vi "test_Set and Get 9228.vi"(8 "error in (no error)":errorcluster, 11 "TestCase in":refnum<class "Scan Engine Scripting API Custom Device Unit Tests.lvclass">) -> (0 "error out":errorcluster, 3 "TestCase out":refnum<class "Scan Engine Scripting API Custom Device Unit Tests.lvclass">)   [LabVIEW 2017, in "Scan Engine Scripting API Custom Device Unit Tests.lvclass"]
uses:
  Scan Engine Scripting API Custom Device Unit Tests.lvclass
  Scan Engine Scripting API Custom Device Unit Tests.lvclass/Scan Engine Scripting API Custom Device Unit Tests.ctl
  8367f121-9304-47f9-89de-0b88beeae42b.vi
  Utility/Set Error.vi
  <vilib>/Utility/error.llb/Clear Errors.vi
  Scripting/Modules/NI 9228/NI 9228.lvclass
  C:/Users/nitest/Documents/niveristand-scan-engine-ethercat-custom-device/Custom Device Source/Scripting/Modules/Module/Module.lvclass
  Modules.lvlibp/SD Module/SD Module.lvclass
  C:/Users/nitest/Documents/niveristand-scan-engine-ethercat-custom-device/Custom Device Source/Modules.lvlibp/RSI Module/RSI Module.lvclass
  Scripting/Modules/NI 9224/NI 9224.lvclass
  Modules.lvlibp/RSI Module/Read Module Page Property.vi
  Modules.lvlibp/RSI Module/Read Model.vi
  Scripting/Utility/Convert Module Model to Module Class.vi
  Modules.lvlibp/SD Module/Read DIO mode.vi
  Modules.lvlibp/RSI Module/Read Channels.vi
  Scripting/Utility/Convert to DI Module.vi
  Scripting/Utility/Convert to DO Module.vi
  Scripting/Utility/Convert to CI PWM Module.vi
  Scripting/Utility/Convert to CDO Module.vi
  Scripting/Utility/Convert to PWM Module.vi
  Globals/Error Strings.vi
  Scripting/Utility/Convert to AI Vrms Module.vi
  Scripting/Utility/Convert to AI Module.vi
  Scripting/Modules/Module/Module.lvclass
  Modules.lvlibp/9224/9224.lvclass
  <vilib>/addons/_JKI Toolkits/VI Tester/TestCase.llb/TestCase.lvclass
  Scripting/Scan Engine Scripting.lvlib
  C:/Program Files (x86)/National Instruments/LabVIEW 2017/vi.lib/addons/_JKI Toolkits/VI Tester/TestCase.llb/TestCase.lvclass
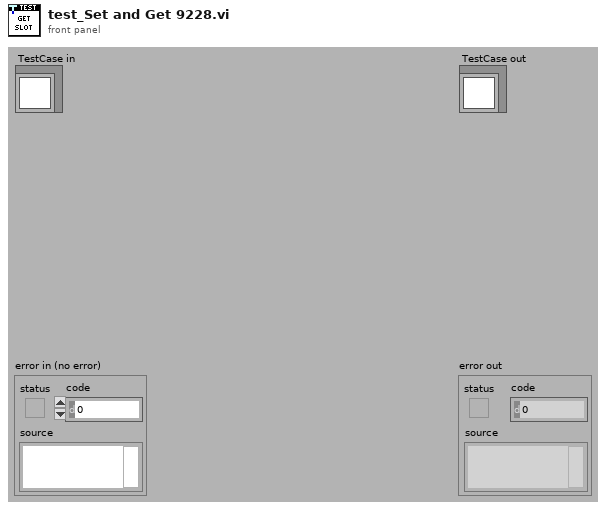
[diagram p1: front panel]
types:
  T1 = typedef "Custom Device API.lvlib/Custom Device Item Ref.ctl" = u64
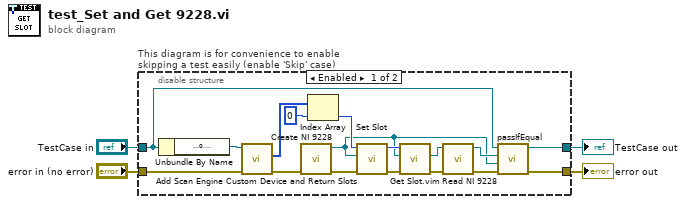
[diagram p0: block diagram]
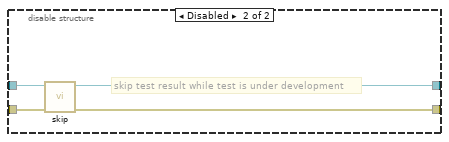
[diagram p2: hidden frame]
diagram:
  n1 = disable-structure "This diagram is for convenience to enable skipping a test easily (enable 'Skip' case)" shown="Enabled" {
    disable-tunnel: "TestCase in" -> [w18 w25]
    disable-tunnel: [w12 w23] -> w1
    disable-tunnel: [w16 w24] -> w3
    disable-tunnel: "error in (no error)" -> [w5 w22]
    frame Enabled {
      n2 = Unbundle By Name(w18) -> ("target ref"=w8:refnum<k24>)
      n3 = call "Add Scan Engine Custom Device and Return Slots.vi"("error in"=w5, "target ref in"=w8) -> ("error out"=w6:errorcluster, "slot refs"=w7:T1[])  [unwired: 7 in, 1 out]
      n4 = call "Create NI 9228.vi"("error in"=w6) -> ("error out"=w17:errorcluster, "NI 9228 out"=w11:refnum<class "NI 9228.lvclass">)  [unwired: 9 in]
      n5 = Index Array(array=w7, index=0) -> (element=w21:T1)
      n6 = call "Set Slot.vi"("error in"=w17, "module"=w11, "slot ref in"=w21) -> ("error out"=w19:errorcluster, "slot ref out"=w13:T1)  [unwired: 7 in]
      n7 = call "Get Slot.vim"("error in"=w19, "module in"=w11, "slot ref in"=w13) -> ("error out"=w9:errorcluster, "module"=w10:refnum<class "NI 9228.lvclass">)  [unwired: 5 in, 2 out]
      n8 = call "Read NI 9228.vi"("error in"=w9, "NI 9228 in"=w10) -> ("error out"=w14:errorcluster, "NI 9228 out"=w15:refnum<class "NI 9228.lvclass">)  [unwired: 6 in, 2 out]
      n9 = call-dynamic "passIfEqual.vi"("error in (no error)"=w14, "y"=w11, "x"=w15, "TestCase in"=w18) -> ("error out"=w16:errorcluster, "TestCase out"=w12:refnum<class "Scan Engine Scripting API Custom Device Unit Tests.lvclass">)  [unwired: 6 in]
    }
    frame Disabled {
      # "skip test result while test is under development"
      n10 = call <vilib>:"skip.vi"("error in (no error)"=w22, "TestCase in"=w25) -> ("error out"=w24:errorcluster, "TestCase out"=w23:refnum<class "Scan Engine Scripting API Custom Device Unit Tests.lvclass">)  [unwired: 8 in]
    }
  }
  "error out" <- w3
  "TestCase out" <- w1
